vi "Edit cell at coordinates.vi"(9 "Cell Position":T1, 10 "Bounds":T2, 11 "D_Datagrid in":refnum<class "D_Datagrid.lvclass">) -> ()   [LabVIEW 2020, in "D Datagrid Library.lvlib" / "D_Datagrid.lvclass"]
doc: "Launches the EditValue VI for the object located at the specified coordinates."
uses:
  D_Datagrid.lvclass
  <vilib>/Utility/miscctls.llb/LVRectTypeDef.ctl
  <vilib>/Utility/miscctls.llb/LVRowAndColumnTypeDef.ctl
  DatagridElement/DatagridElement.lvclass
  D_Datagrid.lvclass/D_Datagrid.ctl
  DatagridElement/DatagridElement.lvclass/DatagridElement.ctl
  D Datagrid Update Element.ctl
  Write DataElements.vi
  Read DataElements.vi
  DatagridElement/Read Enabled state.vi
  Read Auto update indicator.vi
  Redraw full indicator.vi
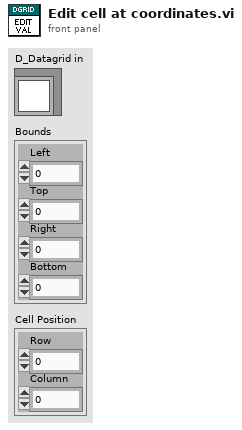
[diagram p1: front panel]
types:
  T1 = typedef "LVRowAndColumnTypeDef.ctl" = cluster{"Row":i32, "Column":i32}
  T2 = typedef "LVRectTypeDef.ctl" = cluster{"Left":i16, "Top":i16, "Right":i16, "Bottom":i16}
  T3 = enum8{"Enabled", "Disabled", "Disabled and Grayed Out"}
  T4 = typedef "D Datagrid Library.lvlib/D_Datagrid.lvclass/D Datagrid Update Element.ctl" = cluster{"Row":i32, "Column":i32, "Element NewVal":refnum<class "DatagridElement.lvclass">, "Element OldVal":refnum<class "DatagridElement.lvclass">, "Changed?":bool}
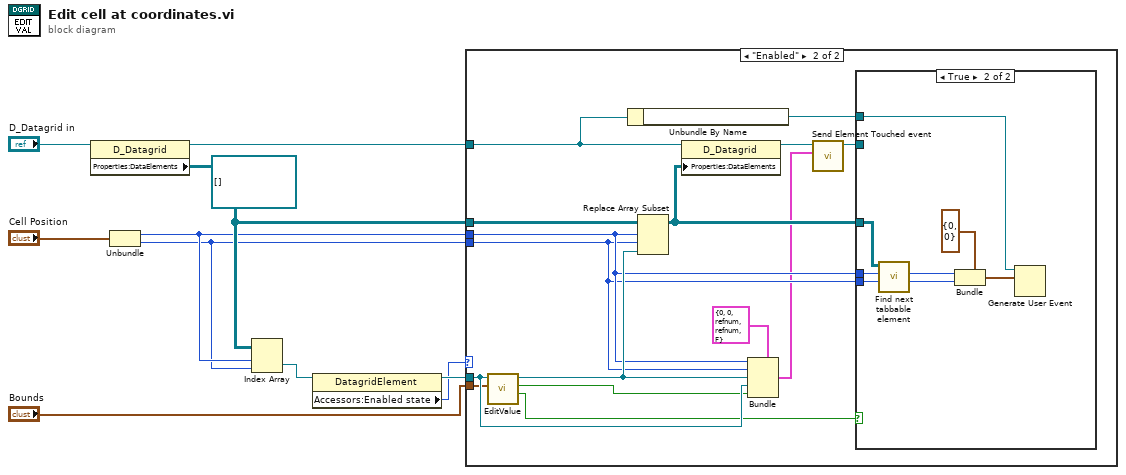
[diagram p0: block diagram]
diagram:
  (unwired) refnum<class "DatagridElement.lvclass">[][] [] ("DataElements")
  n1 = property class="D_Datagrid"(reference="D_Datagrid in") -> (reference out=w9:refnum<class "D_Datagrid.lvclass">, "Properties:DataElements"=w10:refnum<class "DatagridElement.lvclass">[][])  [unwired: 1 in, 1 out]
  n2 = Unbundle("Cell Position") -> (w8:i32, w7:i32)
  n3 = Index Array(array=w10, index (row)=w8, index (col)=w7) -> (element=w6:refnum<class "DatagridElement.lvclass">)
  n4 = property class="DatagridElement"(reference=w6) -> (reference out=w5:refnum<class "DatagridElement.lvclass">, "Accessors:Enabled state"=w4:T3)  [unwired: 1 in, 1 out]
  n5 = case shown="\"Enabled\"" w4 {
    tunnel: w10 -> [_ w25]
    tunnel: w9 -> [_ w23]
    tunnel: w8 -> [_ w16]
    tunnel: w7 -> [_ w15]
    tunnel: w5 -> [_ w22]
    tunnel: "Bounds" -> [_ w21]
    frame Default {
    }
    frame "Enabled" {
      n6 = call-dynamic "EditValue.vi"(10:w21, 11:w22) -> (1:w18:bool, 2:w20:bool, 3:w19:refnum<class "DatagridElement.lvclass">)  [unwired: 6 in, 1 out]
      n7 = Unbundle By Name(w23) -> (w17:refnum<user-event>)
      n8 = Replace Array Subset(array=w25, new element=w19, index (row)=w16, index (col)=w15) -> (w14:refnum<class "DatagridElement.lvclass">[][])
      n9 = property class="D_Datagrid"(reference=w23, "Properties:DataElements"=w14) -> (reference out=w13:refnum<class "D_Datagrid.lvclass">)  [unwired: 1 in, 1 out]
      n10 = Bundle(cluster=T4 {"Row"=0, "Column"=0, "Element NewVal"=refnum, "Element OldVal"=refnum, "Changed?"=FALSE} ("event data"), w16, w15, w19, w22, w20) -> (w11:T4)
      n11 = call-dynamic "Send Element Touched event.vi"(10:w11, 11:w13) -> (3:w12:refnum<class "D_Datagrid.lvclass">)  [unwired: 8 in, 1 out]
      n12 = case shown="True" w18 {
        tunnel: w17 -> [_ w33]
        tunnel: w16 -> [_ w30]
        tunnel: w15 -> [_ w29]
        tunnel: w14 -> [_ w28]
        tunnel: w12 -> [_ _]
        frame False {
        }
        frame True {
          n13 = call "Find next tabbable element.vi"(9:w29, 10:w30, 11:w28) -> (1:w26:i32, 2:w27:i32)  [unwired: 7 in]
          n14 = Bundle(cluster=T1 {"Row"=0, "Column"=0} ("event data"), w27, w26) -> (w31:T1)
          n15 = Generate User Event(user event=w33, event data cluster=w31) -> ()  [unwired: 2 in, 2 out]
        }
      }
    }
  }
